vi "OscCapture (SubVI).vi"(7 "IIR":T1={"Topology"=enum."Off", "Type"=enum."Bandpass", "Order"=2, "Lower Fc"=100.0, "Upper Fc"=200.0, "PB Ripple"=1.0, "SB Attenuation"=60.0} {"PB Ripple" format="%0.2f"; "SB Attenuation" format="%0.2f"; "Lower Fc" format="%0.2p"; "Upper Fc" format="%0.2p"}, 8 "error in (no error)":errorcluster, 11 "A5000_param in":T2={"ChannelA"={"Enabled"=FALSE, "Coupling"=0, "Range"=0, "Analogue Offset"=0.0}, "ChannelB"={"Enabled"=FALSE, "Coupling"=0, "Range"=0, "Analogue Offset"=0.0}, "Trigger"={"Trigger Enabled"=FALSE, "Trigger Source"=enum."Channel A", "Trigger Threshold (volts)"=0.0, "Trigger Direction"=0, "Trigger Delay (samples)"=0, "Auto Trigger Time (ms)"=0}, "MaxADCvalue"=0, "handle"=0, "Acquisition"={"preTriggerSamples"=0, "postTriggerSamples"=0, "timebase"=0, "Down-Sample Mode"=0, "Down Sample Ratio"=0}, "Device Info"={"Driver Version"="", "USB Version"="", "Hardware"="", "Variant"="", "Batch and Serial"="", "Cal Date"="", "Kernel Version"="", "Digital HW Version"="", "Analogue HW Version"="", "MSO"=FALSE, "Number of channels"=0}, "Properties"={"Sample Frequency"=0.0, "Sample Rate"=0.0, "Max Samples Available"=0, "Number of Samples"=0, "Total Capture Time (sec) "=0.0, "Max Total Capture Time Available (sec)"=0.0}, "Resolution"=0, "EmulateV"=FALSE, "General AWG Settings"={"Peak-to-Peak Voltage (microvolts)"=2000000, "Offset Voltage (microvolts)"=0, "Wave Type"=0, "Sweep Type"=0, "Shots"=0, "Sweeps"=0, "Trigger Type"=0, "Trigger Source"=0, "Ext. Threshold (ADC count)"=0, "White Noise/PRBS"=0}, "Standard Waveform Settings"={"Start Frequency"=1000.0, "Stop Frequency"=1000.0, "Increment"=0.0, "Dwell Time (seconds)"=0.0}, "Arbitrary Waveform Settings"={"Arbirary waveform file path"=path "", "Index Mode"=0}, "AutoDiapChA"=FALSE, "AutoDiapChB"=FALSE} {"Arbitrary Waveform Settings"."Index Mode" items=["Single", "Dual", "Quad"]; "Standard Waveform Settings"."Stop Frequency" min=0.03 max=1000000.0; "Standard Waveform Settings"."Start Frequency" min=0.03 max=1000000.0; "General AWG Settings"."White Noise/PRBS" items=["Normal", "White Noise", "PRBS"]; "General AWG Settings"."Trigger Source" items=["None", "Scope Trigger", "Aux. In", "Ext. In", "Software Trigger"]; "General AWG Settings"."Trigger Type" items=["Rising", "Falling", "Gate High", "Gate Low"]; "General AWG Settings"."Sweep Type" items=["Up", "Down", "Up-Down", "Down-Up"]; "General AWG Settings"."Wave Type" items=["Sine", "Square", "Triangle", "Ramp Up", "Ramp Down", "Sinc", "Gaussian", "Half Sine", "DC", "Arbitrary"]; "Resolution" items=["8-bit", "12-bit", "14-bit", "15-bit (max. 2 ch.)", "16-bit (max. 1 ch.)"]; "Properties"."Max Total Capture Time Available (sec)" format="%.3p"; "Properties"."Sample Frequency" format="%.3p"; "Properties"."Sample Rate" format="%.3p"; "Properties"."Max Samples Available" format="%.3p"; "Properties"."Total Capture Time (sec)" format="%.3p"; "Acquisition"."Down Sample Ratio" min=1 step=1; "Acquisition"."Down-Sample Mode" items=["None"=0, "Aggregate"=1, "Decimate"=2, "Average"=4]; "Trigger"."Trigger Direction" items=["Rising"=2, "Falling"=3]; "ChannelB"."Range" items=["10 mV", "20 mV", "50 mV", "100 mV", "200 mV", "500 mV", "1 V", "2 V", "5 V", "10 V", "20 V"]; "ChannelB"."Coupling" items=["AC", "DC"]; "ChannelA"."Range" items=["10 mV", "20 mV", "50 mV", "100 mV", "200 mV", "500 mV", "1 V", "2 V", "5 V", "10 V", "20 V"]; "ChannelA"."Coupling" items=["AC", "DC"]}) -> (0 "error out":errorcluster, 1 "noOfSamples":u32, 2 "Array":waveform(dbl)[](array[waveform]), 3 "A5000_param out":T2={"ChannelA"={"Enabled"=FALSE, "Coupling"=0, "Range"=0, "Analogue Offset"=0.0}, "ChannelB"={"Enabled"=FALSE, "Coupling"=0, "Range"=0, "Analogue Offset"=0.0}, "Trigger"={"Trigger Enabled"=FALSE, "Trigger Source"=enum."Channel A", "Trigger Threshold (volts)"=0.0, "Trigger Direction"=0, "Trigger Delay (samples)"=0, "Auto Trigger Time (ms)"=0}, "MaxADCvalue"=0, "handle"=0, "Acquisition"={"preTriggerSamples"=0, "postTriggerSamples"=0, "timebase"=0, "Down-Sample Mode"=0, "Down Sample Ratio"=0}, "Device Info"={"Driver Version"="", "USB Version"="", "Hardware"="", "Variant"="", "Batch and Serial"="", "Cal Date"="", "Kernel Version"="", "Digital HW Version"="", "Analogue HW Version"="", "MSO"=FALSE, "Number of channels"=0}, "Properties"={"Sample Frequency"=0.0, "Sample Rate"=0.0, "Max Samples Available"=0, "Number of Samples"=0, "Total Capture Time (sec) "=0.0, "Max Total Capture Time Available (sec)"=0.0}, "Resolution"=0, "EmulateV"=FALSE, "General AWG Settings"={"Peak-to-Peak Voltage (microvolts)"=2000000, "Offset Voltage (microvolts)"=0, "Wave Type"=0, "Sweep Type"=0, "Shots"=0, "Sweeps"=0, "Trigger Type"=0, "Trigger Source"=0, "Ext. Threshold (ADC count)"=0, "White Noise/PRBS"=0}, "Standard Waveform Settings"={"Start Frequency"=1000.0, "Stop Frequency"=1000.0, "Increment"=0.0, "Dwell Time (seconds)"=0.0}, "Arbitrary Waveform Settings"={"Arbirary waveform file path"=path "", "Index Mode"=0}, "AutoDiapChA"=FALSE, "AutoDiapChB"=FALSE} {"Arbitrary Waveform Settings"."Index Mode" items=["Single", "Dual", "Quad"]; "Standard Waveform Settings"."Stop Frequency" min=0.03 max=1000000.0; "Standard Waveform Settings"."Start Frequency" min=0.03 max=1000000.0; "General AWG Settings"."White Noise/PRBS" items=["Normal", "White Noise", "PRBS"]; "General AWG Settings"."Trigger Source" items=["None", "Scope Trigger", "Aux. In", "Ext. In", "Software Trigger"]; "General AWG Settings"."Trigger Type" items=["Rising", "Falling", "Gate High", "Gate Low"]; "General AWG Settings"."Sweep Type" items=["Up", "Down", "Up-Down", "Down-Up"]; "General AWG Settings"."Wave Type" items=["Sine", "Square", "Triangle", "Ramp Up", "Ramp Down", "Sinc", "Gaussian", "Half Sine", "DC", "Arbitrary"]; "Resolution" items=["8-bit", "12-bit", "14-bit", "15-bit (max. 2 ch.)", "16-bit (max. 1 ch.)"]; "Properties"."Max Total Capture Time Available (sec)" format="%.3p"; "Properties"."Sample Frequency" format="%.3p"; "Properties"."Sample Rate" format="%.3p"; "Properties"."Max Samples Available" format="%.3p"; "Properties"."Total Capture Time (sec)" format="%.3p"; "Acquisition"."Down Sample Ratio" min=1 step=1; "Acquisition"."Down-Sample Mode" items=["None"=0, "Aggregate"=1, "Decimate"=2, "Average"=4]; "Trigger"."Trigger Direction" items=["Rising"=2, "Falling"=3]; "ChannelB"."Range" items=["10 mV", "20 mV", "50 mV", "100 mV", "200 mV", "500 mV", "1 V", "2 V", "5 V", "10 V", "20 V"]; "ChannelB"."Coupling" items=["AC", "DC"]; "ChannelA"."Range" items=["10 mV", "20 mV", "50 mV", "100 mV", "200 mV", "500 mV", "1 V", "2 V", "5 V", "10 V", "20 V"]; "ChannelA"."Coupling" items=["AC", "DC"]}, 5 "overflow":i16)   [LabVIEW 2017]
uses:
  controls/A5000_param.ctl
  <vilib>/measure/macond.llb/IIR Filter for N Chan.vi
  <vilib>/measure/NI_MAPro.lvlib
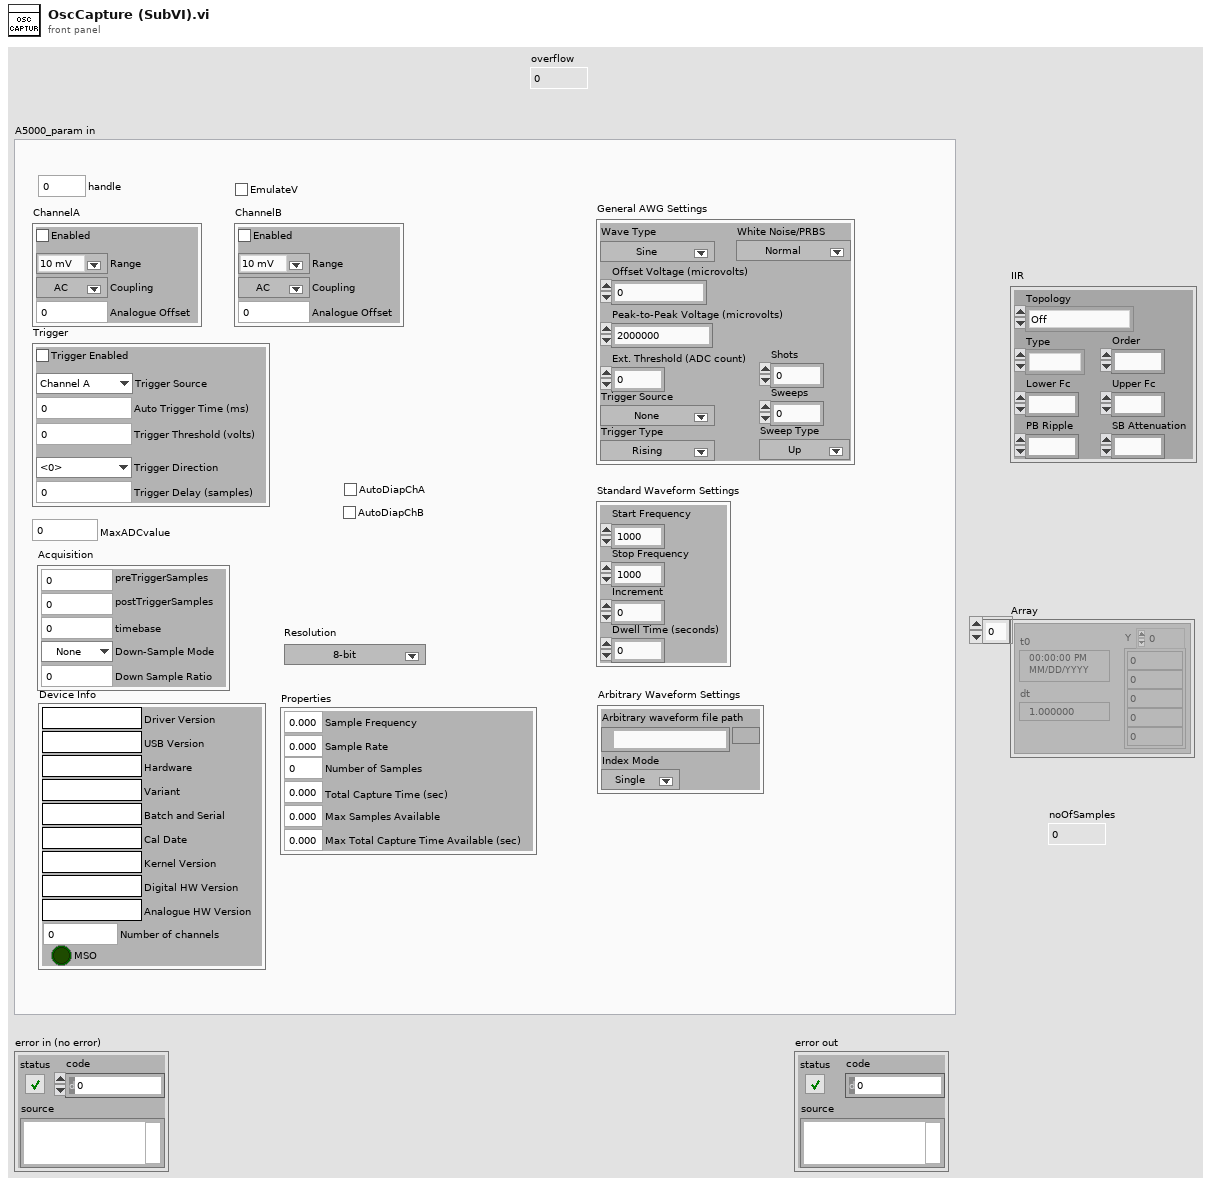
[diagram p1: front panel]
types:
  T1 = cluster{"Topology":enum16{"Off", "Butterworth", "Chebyshev", "Inverse Chebyshev", "Elliptic", "Bessel"}, "Type":enum16{"Lowpass", "Highpass", "Bandpass", "Bandstop"}, "Order":i32, "Lower Fc":dbl, "Upper Fc":dbl, "PB Ripple":dbl, "SB Attenuation":dbl}
  T2 = typedef "A5000_param.ctl" = cluster{"ChannelA":cluster{"Enabled":bool, "Coupling":i16, "Range":u16, "Analogue Offset":sgl}, "ChannelB":cluster{"Enabled":bool, "Coupling":i16, "Range":u16, "Analogue Offset":sgl}, "Trigger":cluster{"Trigger Enabled":bool, "Trigger Source":enum16{"Channel A", "Channel B", "Channel C", "Channel D", "Ext."}, "Trigger Threshold (volts)":dbl, "Trigger Direction":u16, "Trigger Delay (samples)":u32, "Auto Trigger Time (ms)":i16}, "MaxADCvalue":i16, "handle":i16, "Acquisition":cluster{"preTriggerSamples":i32, "postTriggerSamples":i32, "timebase":u32, "Down-Sample Mode":u32, "Down Sample Ratio":u32}, "Device Info":cluster{"Driver Version":string, "USB Version":string, "Hardware":string, "Variant":string, "Batch and Serial":string, "Cal Date":string, "Kernel Version":string, "Digital HW Version":string, "Analogue HW Version":string, "MSO":bool, "Number of channels":i16}, "Properties":cluster{"Sample Frequency":sgl, "Sample Rate":sgl, "Max Samples Available":i32, "Number of Samples":u32, "Total Capture Time (sec) ":sgl, "Max Total Capture Time Available (sec)":sgl}, "Resolution":i32, "EmulateV":bool, "General AWG Settings":cluster{"Peak-to-Peak Voltage (microvolts)":u32, "Offset Voltage (microvolts)":i32, "Wave Type":u32, "Sweep Type":u32, "Shots":u32, "Sweeps":u32, "Trigger Type":u32, "Trigger Source":u32, "Ext. Threshold (ADC count)":i16, "White Noise/PRBS":u32}, "Standard Waveform Settings":cluster{"Start Frequency":dbl, "Stop Frequency":dbl, "Increment":dbl, "Dwell Time (seconds)":dbl}, "Arbitrary Waveform Settings":cluster{"Arbirary waveform file path":path, "Index Mode":u32}, "AutoDiapChA":bool, "AutoDiapChB":bool}
  T3 = cluster{"preTriggerSamples":i32, "postTriggerSamples":i32, "timebase":u32, "Down-Sample Mode":u32, "Down Sample Ratio":u32}
  T4 = cluster{"Enabled":bool, "Coupling":i16, "Range":u16, "Analogue Offset":sgl}
  T5 = cluster{"Driver Version":string, "USB Version":string, "Hardware":string, "Variant":string, "Batch and Serial":string, "Cal Date":string, "Kernel Version":string, "Digital HW Version":string, "Analogue HW Version":string, "MSO":bool, "Number of channels":i16}
  T6 = cluster{"Trigger Enabled":bool, "Trigger Source":enum16{"Channel A", "Channel B", "Channel C", "Channel D", "Ext."}, "Trigger Threshold (volts)":dbl, "Trigger Direction":u16, "Trigger Delay (samples)":u32, "Auto Trigger Time (ms)":i16}
  T7 = cluster{"Sample Frequency":sgl, "Sample Rate":sgl, "Max Samples Available":i32, "Number of Samples":u32, "Total Capture Time (sec) ":sgl, "Max Total Capture Time Available (sec)":sgl}
  T8 = cluster{"Channel D Buffer":i16[], "Channel C Buffer":i16[], "Channel B Buffer":i16[], "Channel A Buffer":i16[], "Port 0 Max Buffer":i32[], "Port 1 Max Buffer":i32[]}
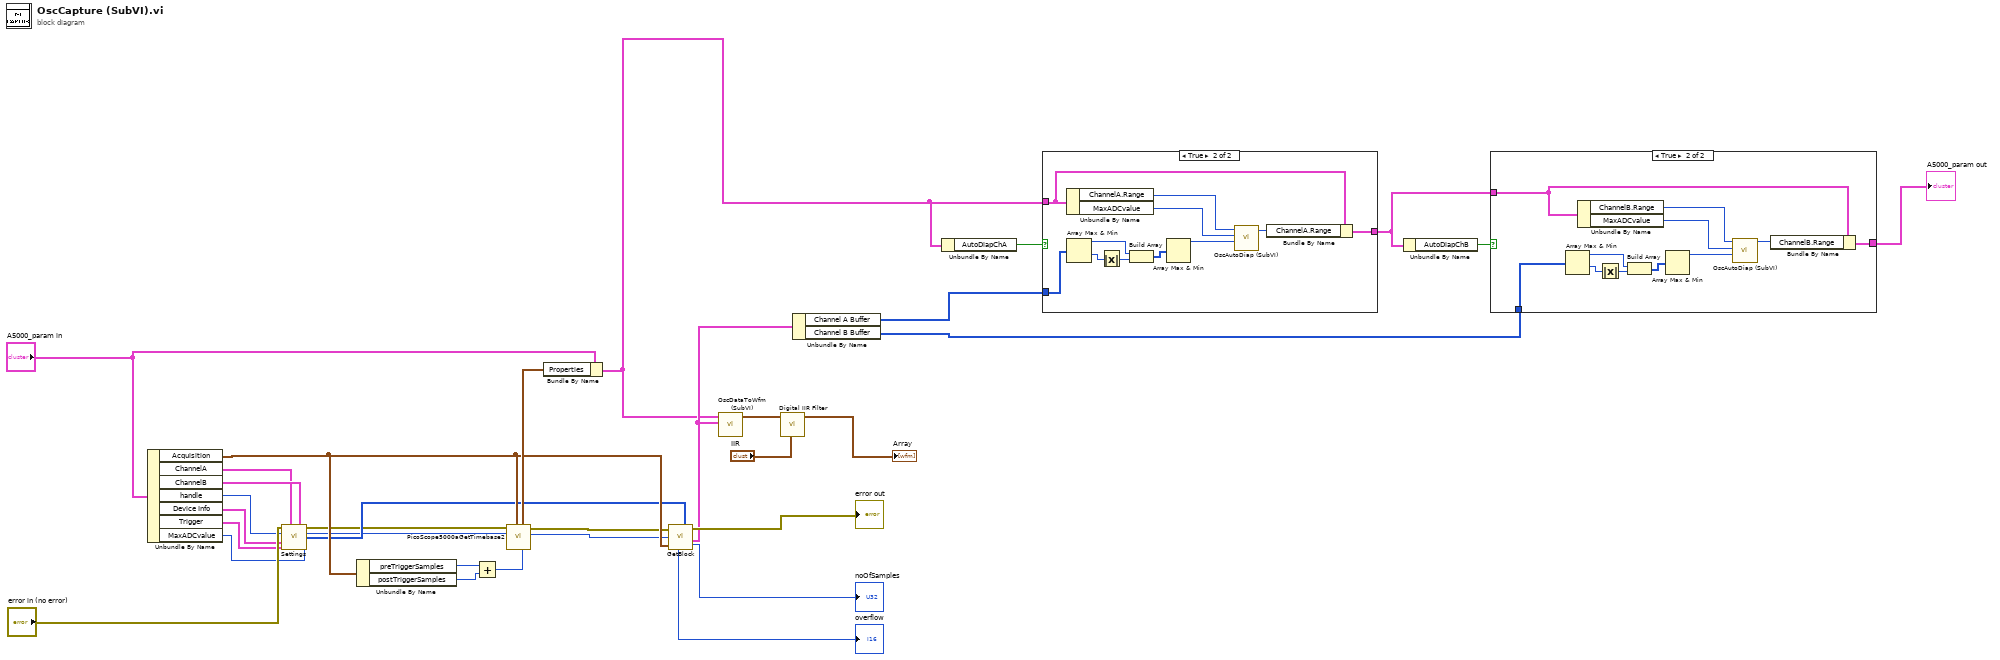
[diagram p0: block diagram]
diagram:
  n1 = Unbundle By Name("A5000_param in") -> ("Acquisition"=w29:T3, "ChannelA"=w23:T4, "ChannelB"=w24:T4, "handle"=w25:i16, "Device Info"=w26:T5, "Trigger"=w27:T6, "MaxADCvalue"=w28:i16)
  n2 = call "Settings.vi"("error in"="error in (no error)", "Channel A Settings"=w23, "Channel B Settings"=w24, "handle in"=w25, "Device Info"=w26, "Trigger Settings"=w27, "Max ADC value"=w28) -> ("error out"=w12:errorcluster, "handle out"=w14:i16, "enabled array"=w16:i16[])  [unwired: 6 in]
  n3 = Unbundle By Name(w29) -> ("preTriggerSamples"=w17:i32, "postTriggerSamples"=w18:i32)
  n4 = Add(x=w17, y=w18) -> (x+y=w19:i32)
  n5 = call "PicoScope5000aGetTimebase2.vi"("Number of Samples"=w19, "Acquisition Settings"=w29, "handle in"=w14, "error in (no error)"=w12) -> ("handle out"=w15:i16, "error out"=w13:errorcluster, "Properties Panel"=w30:T7)  [unwired: 5 in]
  n6 = Bundle By Name(cluster="A5000_param in", "Properties"=w30) -> (w6:T2)
  n7 = call "GetBlock.vi"("error in"=w13, "handle in"=w15, "Acquisition Settings"=w29, "enabled array"=w16) -> ("overflow"=→"overflow":i16, "error IO"=→"error out":errorcluster, "noOfSamples"=→"noOfSamples":u32, "Buffers (Max or non-aggregated)"=w8:T8)  [unwired: 1 in, 2 out]
  n8 = call "OscDataToWfm (SubVI).vi"("Data"=w8, "A5000_param"=w6) -> ("Array"=w9:waveform(dbl)[])  [unwired: 9 in]
  n9 = call-poly <vilib>:"Digital IIR Filter.vi"("IIR filter specifications"="IIR", "signal(s) in"=w9) -> ("signal(s) out"=→"Array":waveform(dbl)[])  [unwired: 7 in, 2 out]
  n10 = Unbundle By Name(w8) -> ("Channel A Buffer"=w7:i16[], "Channel B Buffer"=w4:i16[])
  n11 = Unbundle By Name(w6) -> ("AutoDiapChA"=w5:bool)
  n12 = case shown="True" w5 {
    tunnel: w7 -> [_ w40]
    tunnel: w6 -> [w33 w35]
    tunnel: [w33 w34] -> w2
    frame False {
    }
    frame True {
      n13 = Unbundle By Name(w35) -> ("ChannelA.Range"=w37:u16, "MaxADCvalue"=w39:i16)
      n14 = Array Max & Min(array=w40) -> (max value=w42:i16, min value=w44:i16)  [unwired: 2 out]
      n15 = Absolute Value(x=w44) -> (abs(x)=w43:i16)
      n16 = Build Array(w42, w43) -> (w41:i16[])
      n17 = Array Max & Min(array=w41) -> (max value=w38:i16)  [unwired: 3 out]
      n18 = call "OscAutoDiap (SubVI).vi"("Numeric"=w38, "MaxADCvalue"=w39, "Range"=w37) -> ("y"=w36:i16)  [unwired: 8 in]
      n19 = Bundle By Name(cluster=w35, "ChannelA.Range"=w36) -> (w34:T2)
    }
  }
  n20 = Unbundle By Name(w2) -> ("AutoDiapChB"=w3:bool)
  n21 = case shown="True" w3 {
    tunnel: w4 -> [_ w48]
    tunnel: w2 -> [w45 w47]
    tunnel: [w45 w46] -> w1
    frame False {
    }
    frame True {
      n22 = Array Max & Min(array=w48) -> (max value=w54:i16, min value=w56:i16)  [unwired: 2 out]
      n23 = Unbundle By Name(w47) -> ("ChannelB.Range"=w50:u16, "MaxADCvalue"=w52:i16)
      n24 = Absolute Value(x=w56) -> (abs(x)=w55:i16)
      n25 = Build Array(w54, w55) -> (w53:i16[])
      n26 = Array Max & Min(array=w53) -> (max value=w51:i16)  [unwired: 3 out]
      n27 = call "OscAutoDiap (SubVI).vi"("Numeric"=w51, "MaxADCvalue"=w52, "Range"=w50) -> ("y"=w49:i16)  [unwired: 8 in]
      n28 = Bundle By Name(cluster=w47, "ChannelB.Range"=w49) -> (w46:T2)
    }
  }
  "A5000_param out" <- w1
